vi "CheesyDrive.vi"(6 "Quickturn":bool, 7 "WheelNonLinearity":dbl=0.65, 8 "negInertiaScalar":dbl=1.0, 9 "Sensitivty":dbl=1.0, 10 "Wheel":dbl(slide) scale=-1.0..1.0, 11 "Throttle":dbl(slide)=0.007874015748031496 scale=-1.0..1.0) -> (2 "Right PWM":dbl, 3 "Left PWM":dbl)   [LabVIEW 2017]
doc: "Implements CheesyDrive. CheesyDrive means that the turn joystick controls the radius of turning instead of the rate of turning. Also implements QuickStop and QuickTurn."
panel:
  in  "CarLikeTurning":bool
  in  "QSMult":dbl=0.5
  in  "Max dx/dt":dbl=7.0
  in  "alpha":dbl=0.1
  out "Waveform Chart":dbl(graph)
  # "Enable to enable"
  # "(for quickstop decay)"
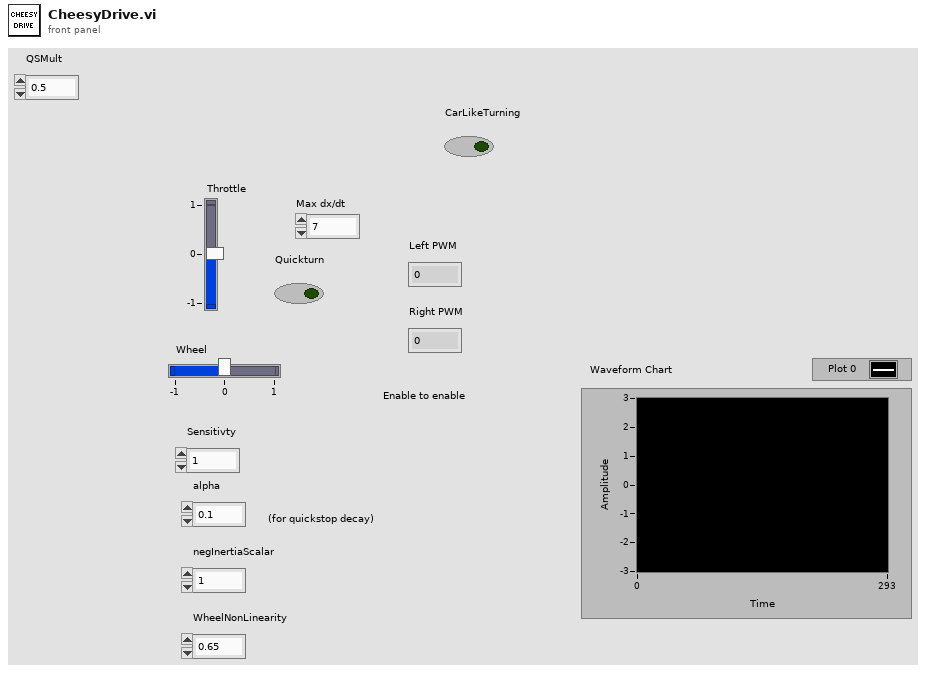
[diagram p1: front panel]
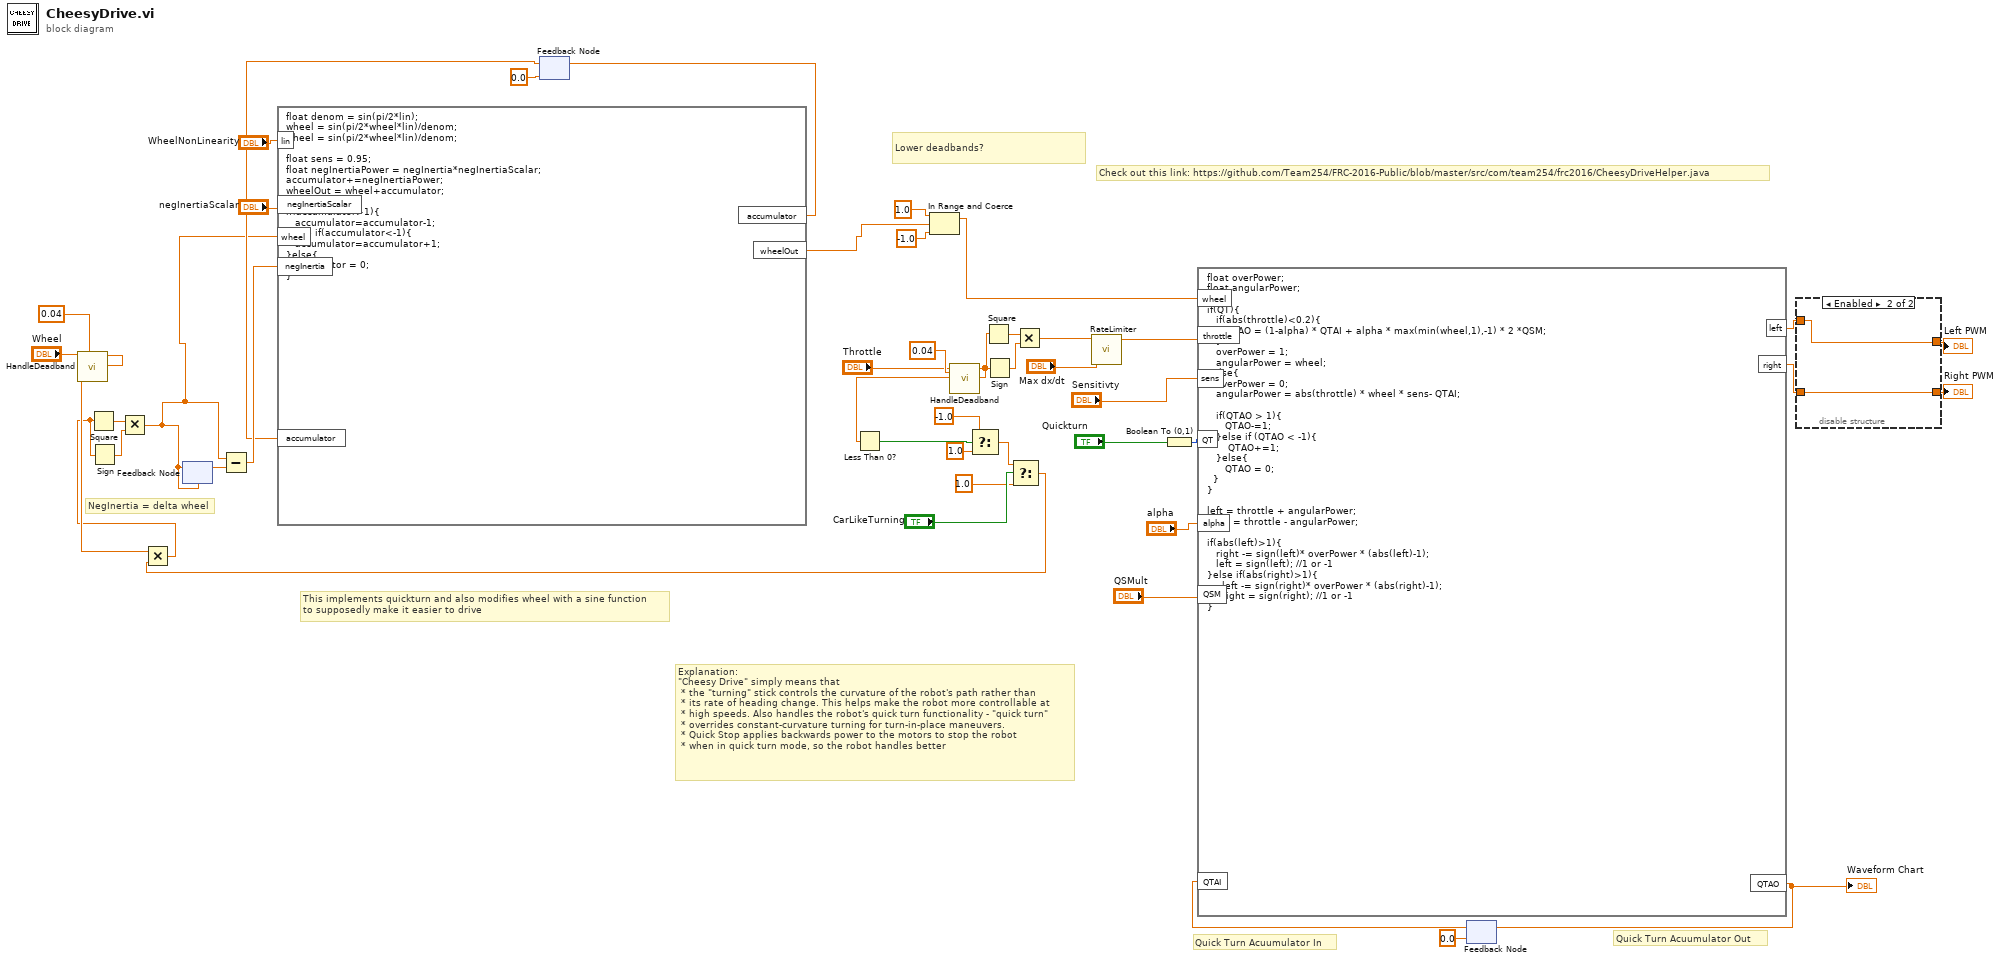
[diagram p0: block diagram]
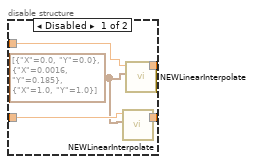
[diagram p2: hidden frame]
diagram:
  # "This implements quickturn and also modifies wheel with a sine function\nto supposedly make it easier to drive"
  # "Lower deadbands?"
  # "NegInertia = delta wheel"
  # "Explanation:\n\"Cheesy Drive\" simply means that\n * the \"turning\" stick controls the curvature of the robot's path rather than\n * its rate of heading change. This helps make the robot more controllable at\n * high speeds. Also handles the robot's quick turn functionality - \"quick turn\"\n * overrides constant-curvature turning for turn-in-place maneuvers.\n * Quick Stop applies backwards power to the motors to stop the robot\n * when in quick turn mode, so the robot handles better"
  # "Quick Turn Acuumulator Out"
  # "Quick Turn Acuumulator In"
  # "Check out this link: https://github.com/Team254/FRC-2016-Public/blob/master/src/com/team254/frc2016/CheesyDriveHelper.java"
  n1 = call "HandleDeadband.vi"("Deadband"=0.04, "Input"="Wheel") -> ("Output"=w7:dbl)  [unwired: 9 in]
  n2 = feedback #1(0.0 ("Wheel")) -> (w25:dbl)
  n3 = call "HandleDeadband.vi"("Deadband"=0.04, "Input"="Throttle") -> ("Output"=w8:dbl)  [unwired: 9 in]
  n4 = Less Than 0?(x=w8) -> (x < 0?=w11:bool)
  n5 = Select(t=-1.0, s=w11, f=1.0) -> (s? t:f=w3:dbl)
  n6 = Square(x=w8) -> (x^2=w36:dbl)
  n7 = Sign(1:w8) -> (0:w35:dbl)
  n8 = Select(t=w3, s="CarLikeTurning", f=1.0) -> (s? t:f=w1:dbl)
  n9 = Multiply(x=w7, y=w1) -> (x*y=w6:dbl)
  n10 = Square(x=w6) -> (x^2=w16:dbl)
  n11 = Sign(1:w6) -> (0:w15:dbl)
  n12 = Multiply(x=w16, y=w15) -> (x*y=w5:dbl)
  n13 = feedback #2(w5) -> (w27:dbl)
  n14 = feedback-in #2(w5) -> ()
  n15 = Subtract(x=w5, y=w27) -> (x-y=w26:dbl)
  n16 = formula code="float denom = sin(pi/2*lin);\nwheel = sin(pi/2*wheel*lin)/denom;\nwheel = sin(pi/2*wheel*lin)/denom;\n\nfloat sens = 0.95;\nfloat negInertiaPower = negInertia*negInertiaScalar;\naccumulator+=negInertiaPower;\nwheelOut = wheel+accumulator;\n\nif(accumulator>1){\n   accumulator=accumulator-1;\n}else if(accumulator<-1){\n   accumulator=accumulator+1;\n}else{\naccumulator = 0;\n}"("wheel"=w5, "negInertia"=w26, "accumulator"=w25, "negInertiaScalar"="negInertiaScalar", "lin"="WheelNonLinearity") -> ("accumulator"=w23:dbl, "wheelOut"=w17:dbl)
  n17 = feedback-in #1(w23) -> ()
  n18 = In Range and Coerce(upper limit=1.0, x=w17, lower limit=-1.0) -> (coerced(x)=w18:dbl)  [unwired: 1 out]
  n19 = Multiply(x=w36, y=w35) -> (x*y=w34:dbl)
  n20 = call "RateLimiter.vi"("Max dx/dt"="Max dx/dt", "Input"=w34) -> ("Output"=w33:dbl)  [unwired: 9 in]
  n21 = Boolean To (0,1)(Boolean="Quickturn") -> (0, 1=w40:i16)
  n22 = feedback #3(0.0 ("QTAccumulatorO")) -> (w38:dbl)
  n23 = formula code="float overPower;\nfloat angularPower;\n\nif(QT){\n   if(abs(throttle)<0.2){\n      QTAO = (1-alpha) * QTAI + alpha * max(min(wheel,1),-1) * 2 *QSM;\n   }\n   overPower = 1;\n   angularPower = wheel;\n}else{\n   overPower = 0;\n   angularPower = abs(throttle) * wheel * sens- QTAI;\n\n   if(QTAO > 1){\n      QTAO-=1;\n   }else if (QTAO < -1){\n       QTAO+=1;\n   }else{\n      QTAO = 0;\n  }\n}\n\nleft = throttle + angularPower;\nright = throttle - angularPower;\n\nif(abs(left)>1){\n   right -= sign(left)* overPower * (abs(left)-1);\n   left = sign(left); //1 or -1\n}else if(abs(right)>1){\n     left -= sign(right)* overPower * (abs(right)-1);\n     right = sign(right); //1 or -1 \n}"("wheel"=w18, "throttle"=w33, "sens"="Sensitivty", "QT"=w40, "alpha"="alpha", "QTAI"=w38, "QSM"="QSMult") -> ("left"=w31:dbl, "right"=w28:dbl, "QTAO"=w41:dbl)
  "Waveform Chart" <- w41
  n24 = feedback-in #3(w41) -> ()
  n25 = disable-structure shown="Enabled" {
    disable-tunnel: w31 -> [w50 w52]
    disable-tunnel: [w49 w52] -> w30
    disable-tunnel: [w48 w51] -> w29
    disable-tunnel: w28 -> [w47 w51]
    frame Disabled {
      w46 = cluster{"X":dbl, "Y":dbl}[] [{"X"=0.0, "Y"=0.0}, {"X"=0.0016, "Y"=0.185}, {"X"=1.0, "Y"=1.0}] ("Points")
      n26 = call "NEWLinearInterpolate.vi"("Points"=w46, "Value"=w47) -> ("Output"=w48:dbl)  [unwired: 9 in]
      n27 = call "NEWLinearInterpolate.vi"("Points"=w46, "Value"=w50) -> ("Output"=w49:dbl)  [unwired: 9 in]
    }
    frame Enabled {
    }
  }
  "Left PWM" <- w30
  "Right PWM" <- w29
